vi "createHealthAndStatus.vi"(8 "error in (no error)":errorcluster, 11 "Boot in":refnum<class "Boot.lvclass">) -> (0 "error out":errorcluster, 2 "HealthAndStatus":refnum<class "RTHealthAndStatus.lvclass">, 3 "Boot out":refnum<class "Boot.lvclass">)   [LabVIEW 2016, in "Boot.lvclass"]
uses:
  Boot.lvclass
  Common_RT_HealthAndStatus/RTHealthAndStatus/RTHealthAndStatus.lvclass
  Resources/HealthAndStatusControlFIFO/HealthAndStatusControlFIFO.lvclass
  D:/Code/ts_M1M3Support/Common_RT_FPGA/IWriteU64FIFO/IWriteU64FIFO.lvclass
  Resources/HealthAndStatusDataFIFO/HealthAndStatusDataFIFO.lvclass
  D:/Code/ts_M1M3Support/Common_RT_FPGA/IReadU32FIFO/IReadU32FIFO.lvclass
  Boot.lvclass/Boot.ctl
  Resources/HealthAndStatusDataFIFO/HealthAndStatusDataFIFO.lvclass/HealthAndStatusDataFIFO.ctl
  Resources/HealthAndStatusControlFIFO/HealthAndStatusControlFIFO.lvclass/HealthAndStatusControlFIFO.ctl
  Common_RT_HealthAndStatus/RTHealthAndStatus/RTHealthAndStatus.lvclass/RTHealthAndStatus.ctl
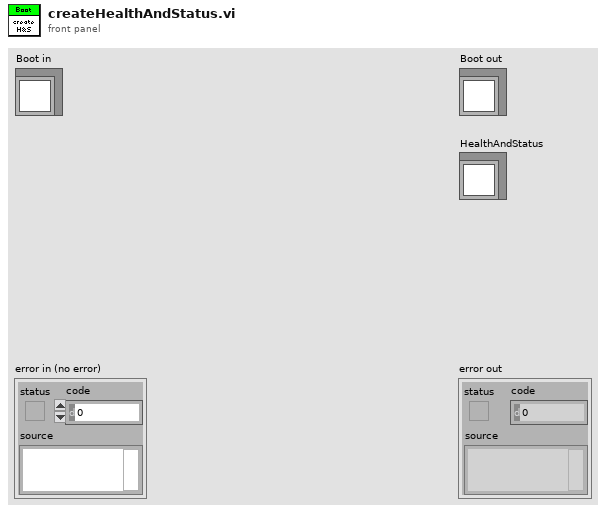
[diagram p1: front panel]
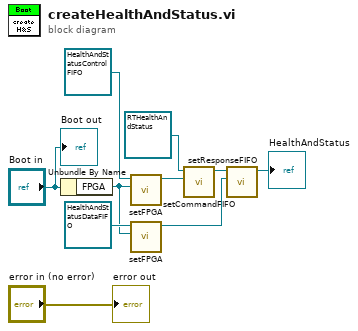
[diagram p0: block diagram]
diagram:
  n1 = Unbundle By Name("Boot in") -> ("FPGA"=w5:refnum<class "FPGA.lvclass">)
  n2 = call "setFPGA.vi"("FPGA"=w5, "HealthAndStatusControlFIFO in"=refnum<class "HealthAndStatusControlFIFO.lvclass"> refnum ("HealthAndStatusControlFIFO.lvclass")) -> ("HealthAndStatusControlFIFO out"=w4:refnum<class "HealthAndStatusControlFIFO.lvclass">)  [unwired: 9 in]
  n3 = call "setFPGA.vi"("FPGA"=w5, "HealthAndStatusDataFIFO in"=refnum<class "HealthAndStatusDataFIFO.lvclass"> refnum ("HealthAndStatusDataFIFO.lvclass")) -> ("HealthAndStatusDataFIFO out"=w3:refnum<class "HealthAndStatusDataFIFO.lvclass">)  [unwired: 9 in]
  n4 = call "setCommandFIFO.vi"("WriteU64FIFO"=w4, "RTHealthAndStatus in"=refnum<class "RTHealthAndStatus.lvclass"> refnum ("RTHealthAndStatus.lvlib:RTHealthAndStatus.lvclass")) -> ("RTHealthAndStatus out"=w9:refnum<class "RTHealthAndStatus.lvclass">)  [unwired: 9 in]
  n5 = call "setResponseFIFO.vi"("ReadU32FIFO"=w3, "RTHealthAndStatus in"=w9) -> ("RTHealthAndStatus out"=→"HealthAndStatus":refnum<class "RTHealthAndStatus.lvclass">)  [unwired: 9 in]
  "error out" <- "error in (no error)"
  "Boot out" <- "Boot in"
